vi "ZipFiles.vi"(1 "Source File/Directory":path, 2 "Target Zip File":path) -> ()   [LabVIEW 2012]
panel:
  out "In Progress":bool
  out "Directory Tree":string(tree)
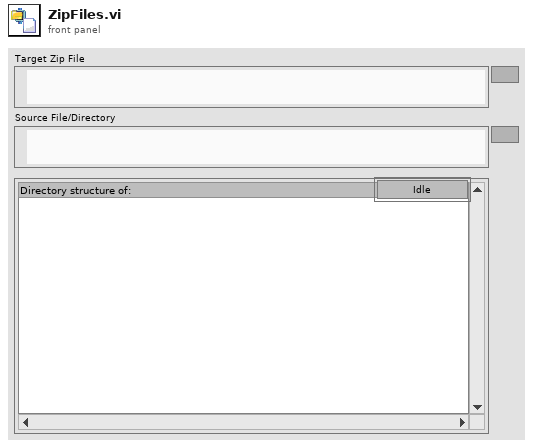
[diagram p1: front panel]
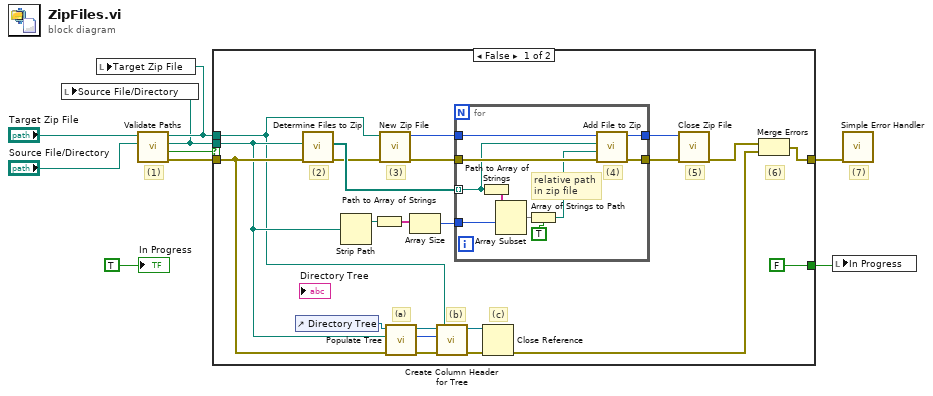
[diagram p0: block diagram]
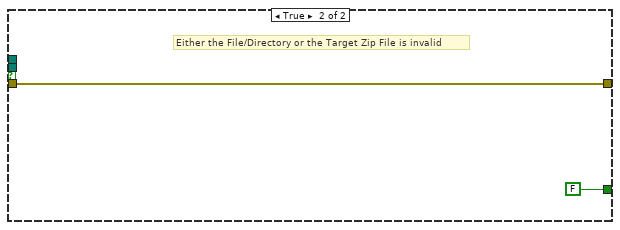
[diagram p2: hidden frame]
diagram:
  # "(7)"
  # "(1)"
  n1 = call "Validate Paths.vi"("File or Directory input"="Source File/Directory", "Target zip file input"="Target Zip File") -> ("error out"=w5:errorcluster, "Invalid Path?"=w6:bool, "File or Directory selected"=w3:path, "Target zip file selected"=w4:path)  [unwired: 6 out]
  n2 = local write "Source File/Directory"(w3) -> ()
  n3 = local write "Target Zip File"(w4) -> ()
  n4 = case shown="False" w6 {
    tunnel: w3 -> [w12 _]
    tunnel: [w22 w43] -> w8
    tunnel: w5 -> [w21 w43]
    tunnel: w4 -> [w11 _]
    tunnel: [FALSE ("In Progress") FALSE ("In Progress")] -> w1
    frame False {
      # "(6)"
      # "(c)"
      # "(b)"
      # "(a)"
      # "(5)"
      # "(3)"
      # "(2)"
      n5 = control-ref of="Directory Tree"() -> (w18:refnum<vi>)
      n6 = call "Determine Files to Zip.vi"("error in (no error)"=w21, "File or Directory"=w12) -> ("error out"=w20:errorcluster, "Array"=w26:path[])  [unwired: 8 out]
      n7 = Strip Path(path=w12) -> (stripped path=w29:path)  [unwired: 1 out]
      n8 = Path to Array of Strings(0:w29) -> (2:w28:string[])  [unwired: 1 out]
      n9 = call <vilib>:"New Zip File.vi"("error in (no error)"=w20, "target"=w11) -> ("error out"=w30:errorcluster, "zip file out"=w31:i64)  [unwired: 1 in, 3 out]
      n10 = call "Populate Tree.vi"("error in (no error)"=w21, "File or Directory"=w12, "Directory Tree"=w18) -> ("error out"=w19:errorcluster, "Number of files found"=w16:i32, "Directory Tree dup"=w17:refnum<vi>)  [unwired: 6 out]
      n11 = Array Size(array=w28) -> (size(s)=w27:i32)
      n12 = call "Create Column Header for Tree.vi"("Target zip file"=w11, "error in (no error)"=w19, "Number of Files Found"=w16, "Directory Tree"=w17) -> ("error out"=w14:errorcluster, "Directory Tree dup"=w15:refnum<vi>)  [unwired: 2 in, 4 out]
      n13 = for {
        tunnel: w26 -> [w39] mode=indexing
        tunnel: w31 -> [w41]
        tunnel: w30 -> [w40]
        tunnel: w27 -> [w37]
        tunnel: [w33] -> w25
        tunnel: [w32] -> w24
        # "(4)"
        # "relative path\nin zip file"
        n14 = Path to Array of Strings(0:w39) -> (2:w38:string[])  [unwired: 1 out]
        n15 = Array Subset(array=w38, index=w37) -> (w36:string[])  [unwired: 1 in]
        n16 = Array of Strings to Path(0:w36, 1:TRUE ("relative")) -> (2:w35:path)
        n17 = call <vilib>:"Add File to Zip.vi"("error in (no error)"=w40, "destination path in zip"=w35, "source file path"=w39, "zip file in"=w41) -> ("error out"=w33:errorcluster, "zip file out"=w32:i64)  [unwired: 6 out]
      }
      n18 = Close Reference(reference=w15, error in (no error)=w14) -> (error out=w13:errorcluster)
      n19 = call <vilib>:"Close Zip File.vi"("error in (no error)"=w25, "zip file in"=w24) -> ("error out"=w23:errorcluster)  [unwired: 1 in, 4 out]
      n20 = Merge Errors(w23, w13) -> (w22:errorcluster)
    }
    frame True {
      # "Either the File/Directory or the Target Zip File is invalid"
    }
  }
  n21 = local write "In Progress"(w1) -> ()
  n22 = call <vilib>:"Simple Error Handler.vi"("error in (no error)"=w8) -> ()  [unwired: 1 in, 8 out]
  "In Progress" <- TRUE ("In Progress")
